vi "validate.vi"(8 "error in":errorcluster, 11 "configuration in":refnum<class "engine configuration.lvclass">) -> (0 "error out":errorcluster, 3 "configuration out":refnum<class "engine configuration.lvclass">)   [LabVIEW 2013, in "engine configuration.lvclass"]
doc: "Provides an interface for performing validation on a given configuration. Any children should define the behavior of this function to ensure that the configuration in memory can be used by the runtime class."
uses:
  engine configuration.lvclass
  <vilib>/NI/Tag Bus Module Framework/root configuration/TBM configuration.lvclass
  engine configuration.lvclass/engine configuration.ctl
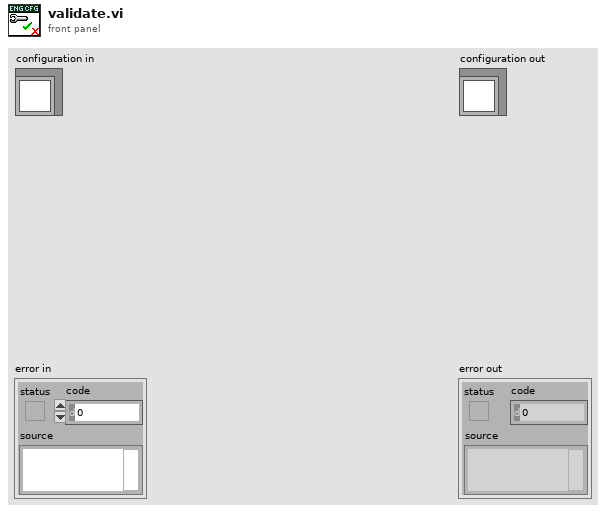
[diagram p1: front panel]
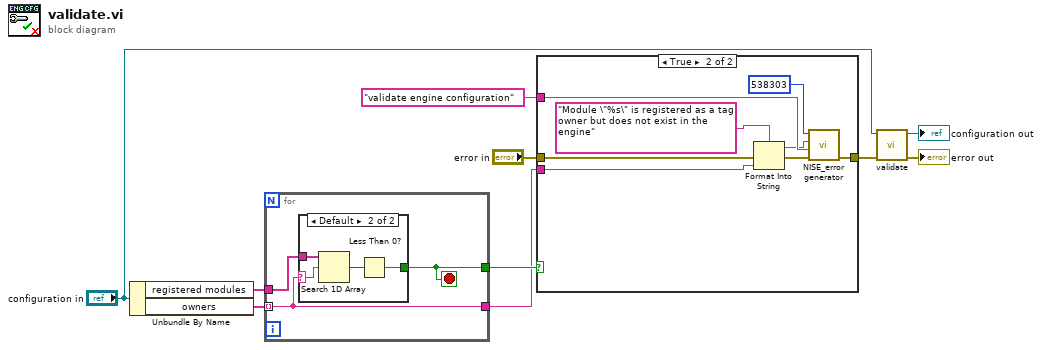
[diagram p0: block diagram]
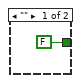
[diagram p3: hidden frame]
diagram:
  n1 = Unbundle By Name("configuration in") -> ("registered modules"=w6:string[], "owners"=w8:string[])
  n2 = for {
    tunnel: w8 -> [w11] mode=indexing
    tunnel: w6 -> [w13]
    tunnel: [w12] -> w7
    tunnel: [w11] -> w4
    stop <- w12 stop-if-true
    n3 = case shown="Default" w11 {
      selector: w11 -> [_ w15]
      tunnel: w13 -> [_ w18]
      tunnel: [FALSE w16] -> w12
      frame "" {
      }
      frame Default {
        n4 = Search 1D Array(1D array=w18, element=w15) -> (index of element=w17:i32)  [unwired: 1 in]
        n5 = Less Than 0?(x=w17) -> (x < 0?=w16:bool)
      }
    }
  }
  n6 = case shown="True" w7 {
    tunnel: "error in" -> [w19 w24]
    tunnel: [w19 w27] -> w1
    tunnel: "validate engine configuration" ("source") -> [_ w25]
    tunnel: w4 -> [_ w21]
    frame False {
    }
    frame True {
      n7 = Format Into String(format string="Module \"%s\" is registered as a tag owner but does not exist in the engine", error in=w24, w21) -> (resulting string=w22:string, error out=w23:errorcluster)  [unwired: 1 in]
      n8 = call <vilib>:"NISE_error generator.vi"("error in"=w23, "source"=w25, "append error message"=w22, "error code (0)"=538303) -> ("error out"=w27:errorcluster)  [unwired: 5 in]
    }
  }
  n9 = call-parent "validate.vi"("error in"=w1, "configuration in"="configuration in") -> ("error out"=→"error out":errorcluster, "configuration out"=→"configuration out":refnum<class "engine configuration.lvclass">)  [unwired: 8 in]
